vi "Robot_Main.vi"() -> ()   [LabVIEW 2013]
uses:
  Support VIs/setpointCluster.ctl
  GainsTDef.ctl
  Support VIs/speeds.ctl
  Support VIs/messageTypes.ctl
  PolarCoordTdef.ctl
  StopTDef.ctl
  <vilib>/robotics/Starter Kit/2.0/9632 Host Interface/NI_Robotics_Starter Kit Host_9632_2.0.lvclass
  <vilib>/robotics/Starter Kit/Host Interface/NI_Robotics_Starter Kit Host.lvclass
panel:
  out "message data":variant
  in  "Polar Coord":T1
  out "message type":T2=enum."Setpoints"
  in  "Speeds":T3
  in  "GainsCluster":T4
  in  "STOP":bool
  in  "Setpoint Cluster":T5
  out "Modulus Setpoint Read":dbl
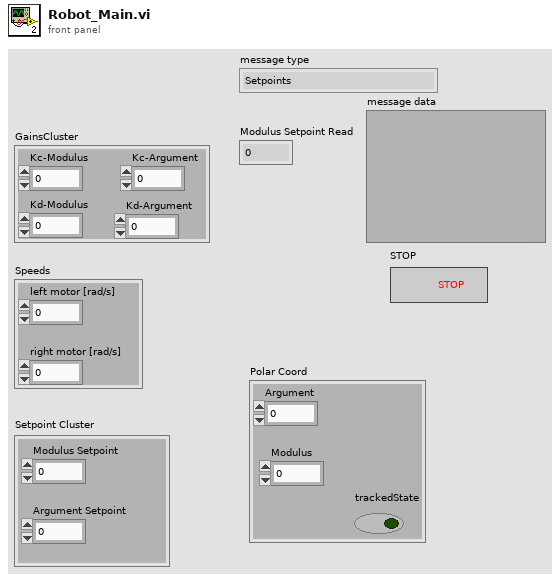
[diagram p1: front panel]
types:
  T1 = typedef "PolarCoordTdef.ctl" = cluster{"Argument":dbl, "Modulus":dbl, "trackedState":bool}
  T2 = typedef "messageTypes.ctl" = enum16{"Speeds", "Stop", "PolarCoordinates", "Gains", "Setpoints"}
  T3 = typedef "speeds.ctl" = cluster{"left motor [rad/s]":dbl, "right motor [rad/s]":dbl}
  T4 = typedef "GainsTDef.ctl" = cluster{"Kc-Modulus":dbl, "Kd-Modulus":dbl, "Kc-Argument":dbl, "Kd-Argument":dbl}
  T5 = typedef "setpointCluster.ctl" = cluster{"Modulus Setpoint":dbl, "Argument Setpoint":dbl}
  T6 = typedef "StopTDef.ctl" = cluster{"stop":bool}
  T7 = typedef "Messages.ctl" = cluster{"message data":variant, "message type":T2}
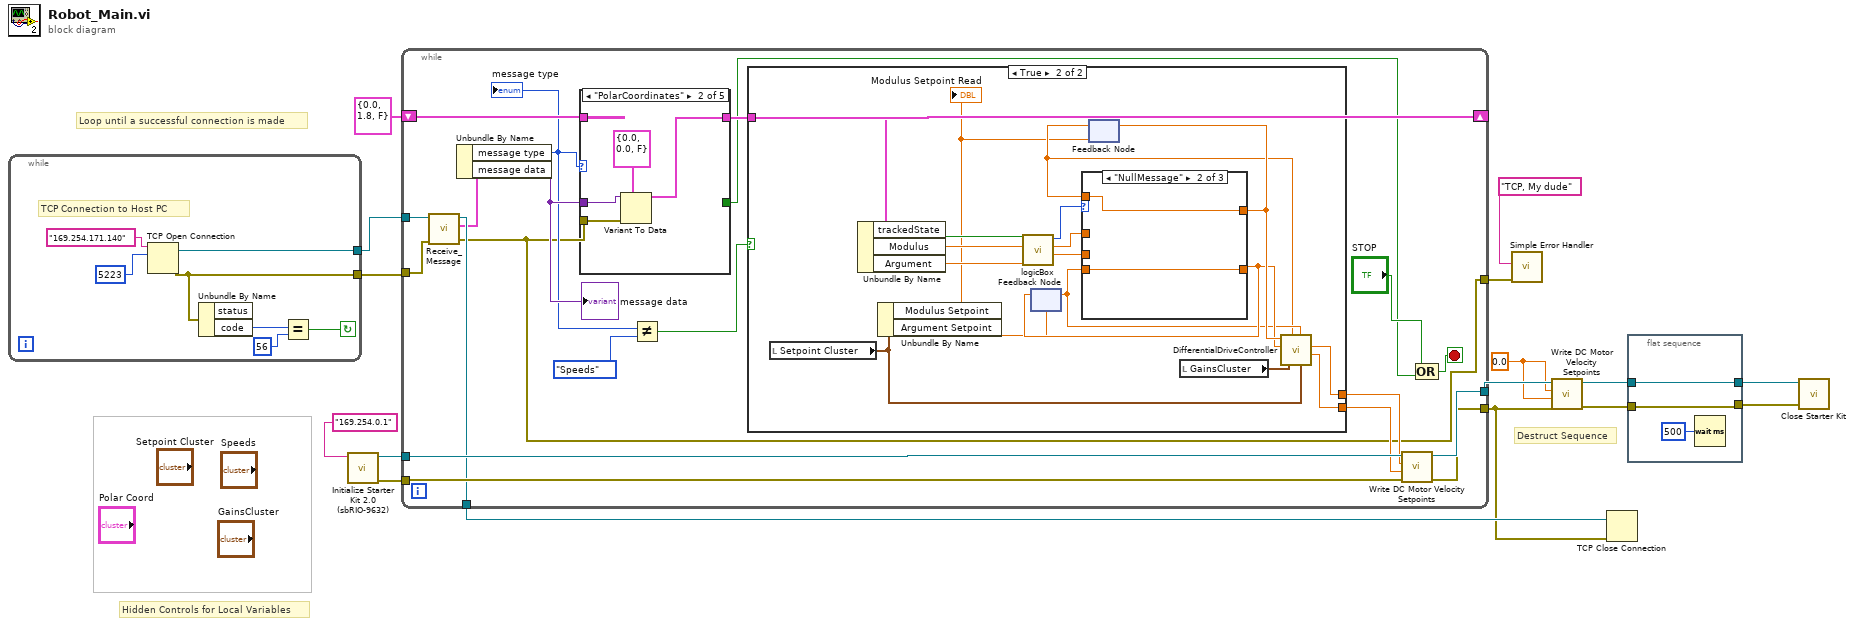
[diagram p0: block diagram]
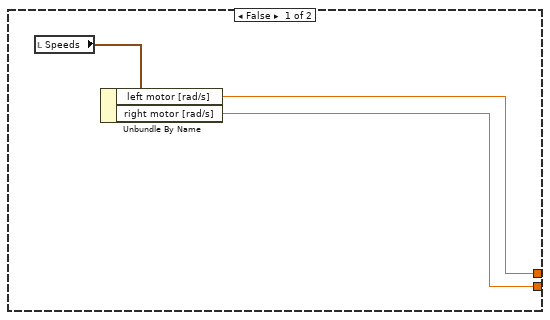
[diagram p2: hidden frame]
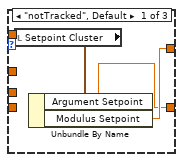
[diagram p3: hidden frame]
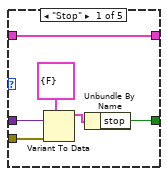
[diagram p5: hidden frame]
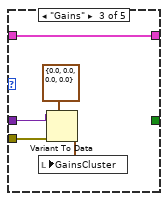
[diagram p6: hidden frame]
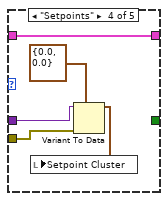
[diagram p7: hidden frame]
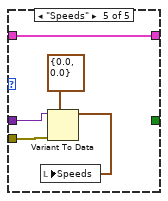
[diagram p8: hidden frame]
diagram:
  w13 = 0.0
  # "Hidden Controls for Local Variables"
  # "Loop until a successful connection is made"
  # "Destruct Sequence"
  n1 = while {
    tunnel: [w23] -> w6
    tunnel: [w20] -> w7
    stop <- w17 continue-if-true
    # "TCP Connection to Host PC"
    n2 = TCP Open Connection(address="169.254.171.140", remote port or service name=u16 5223) -> (connection ID=w23:refnum<k5>, error out=w20:errorcluster)  [unwired: 3 in]
    n3 = Unbundle By Name(w20) -> ("code"=w19:i32)  [unwired: 1 out]
    n4 = Equal?(x=w19, y=56) -> (x = y?=w17:bool)
  }
  n5 = call <vilib>:"Initialize Starter Kit 2.0 (sbRIO-9632).vi"("IP address (\"\")"="169.254.0.1" ("IP address (\"\")")) -> ("error out"=w15:errorcluster, "FPGA starter kit host 2.0 out"=w16:refnum<class "NI_Robotics_Starter Kit Host_9632_2.0.lvclass">)  [unwired: 9 in]
  n6 = while {
    tunnel: w16 -> [w43]
    tunnel: w15 -> [w34]
    tunnel: w7 -> [w39]
    tunnel: [w42] -> w14
    tunnel: [w41] -> w3
    tunnel: w6 -> [w40]
    shift-right: [w38] -> _
    shift-left: T1 {"Argument"=0.0, "Modulus"=1.8, "trackedState"=FALSE} ("Polar Coord") -> [w37]
    tunnel: [w33] -> w4
    tunnel: [w25] -> w2
    stop <- w27 stop-if-true
    n7 = call "Receive_Message.vi"("error in (no error)"=w39, "connection ID IN"=w40) -> ("error out (no error)"=w25:errorcluster, "msg OUT"=w31:T7, "connection ID OUT"=w33:refnum<k5>)  [unwired: 7 in]
    n8 = Unbundle By Name(w31) -> ("message type"=w29:T2, "message data"=w30:variant)
    "message type" <- w29
    "message data" <- w30
    n9 = case shown="\"PolarCoordinates\"" w29 {
      tunnel: w25 -> [w75 w79 w84 w89 w93]
      tunnel: [w73 w78 w83 w88 w95] -> w38
      tunnel: w37 -> [w73 _ w83 w88 w95]
      tunnel: w30 -> [w72 w77 w81 w86 w91]
      tunnel: [w71 _ _ _ _] -> w24
      frame "Stop" {
        n10 = Variant To Data(error in=w75, type=T6 {"stop"=FALSE}, Variant=w72) -> (data=w74:T6)  [unwired: 1 out]
        n11 = Unbundle By Name(w74) -> ("stop"=w71:bool)
      }
      frame "PolarCoordinates" {
        n12 = Variant To Data(error in=w79, type=T1 {"Argument"=0.0, "Modulus"=0.0, "trackedState"=FALSE} ("Polar Coord"), Variant=w77) -> (data=w78:T1)  [unwired: 1 out]
      }
      frame "Gains" {
        n13 = Variant To Data(error in=w84, type=T4 {"Kc-Modulus"=0.0, "Kd-Modulus"=0.0, "Kc-Argument"=0.0, "Kd-Argument"=0.0} ("GainsCluster"), Variant=w81) -> (data=w82:T4)  [unwired: 1 out]
        n14 = local write "GainsCluster"(w82) -> ()
      }
      frame "Setpoints" {
        n15 = Variant To Data(error in=w89, type=T5 {"Modulus Setpoint"=0.0, "Argument Setpoint"=0.0} ("Setpoint Cluster"), Variant=w86) -> (data=w87:T5)  [unwired: 1 out]
        n16 = local write "Setpoint Cluster"(w87) -> ()
      }
      frame "Speeds" {
        n17 = Variant To Data(error in=w93, type=T3 {"left motor [rad/s]"=0.0, "right motor [rad/s]"=0.0} ("Speeds"), Variant=w91) -> (data=w92:T3)  [unwired: 1 out]
        n18 = local write "Speeds"(w92) -> ()
      }
    }
    n19 = Not Equal?(x=w29, y=messageTypes."Speeds") -> (x != y?=w32:bool)
    n20 = case shown="True" w32 {
      tunnel: w38 -> [_ w63]
      tunnel: [w45 w56] -> w36
      tunnel: [w44 w55] -> w35
      frame False {
        n21 = local read "Speeds"() -> (w46:T3)
        n22 = Unbundle By Name(w46) -> ("left motor [rad/s]"=w45:dbl, "right motor [rad/s]"=w44:dbl)
      }
      frame True {
        n23 = local read "Setpoint Cluster"() -> (w48:T5)
        n24 = Unbundle By Name(w63) -> ("trackedState"=w62:bool, "Modulus"=w61:dbl, "Argument"=w60:dbl)
        n25 = Unbundle By Name(w48) -> ("Modulus Setpoint"=w49:dbl, "Argument Setpoint"=w50:dbl)
        "Modulus Setpoint Read" <- w49
        n26 = call "logicBox.vi"("Arg"=w60, "Mod"=w61, "TrackState"=w62) -> ("Arg"=w57:dbl, "Mod"=w58:dbl, "State"=w59:enum16{"notTracked", "NullMessage", "OK"})  [unwired: 6 in]
        n27 = feedback #1(w50) -> (w52:dbl)
        n28 = feedback #2(w49) -> (w51:dbl)
        n29 = case shown="\"NullMessage\"" w59 {
          tunnel: [w65 w67 w69] -> w53
          tunnel: [w66 w68 w70] -> w54
          tunnel: w58 -> [_ _ w70]
          tunnel: w57 -> [_ _ w69]
          tunnel: w51 -> [_ w68 _]
          tunnel: w52 -> [_ w67 _]
          frame "notTracked", Default {
            n30 = local read "Setpoint Cluster"() -> (w64:T5)
            n31 = Unbundle By Name(w64) -> ("Argument Setpoint"=w65:dbl, "Modulus Setpoint"=w66:dbl)
          }
          frame "NullMessage" {
          }
          frame "OK" {
          }
        }
        n32 = feedback-in #1(w53) -> ()
        n33 = feedback-in #2(w54) -> ()
        n34 = local read "GainsCluster"() -> (w47:T4)
        n35 = call "DifferentialDriveController.vi"("Setpoint Cluster"=w48, "prevArgIn"=w52, "GainsCluster"=w47, "prevModIn"=w51, "ArgIn"=w53, "ModIn"=w54) -> ("right motor out"=w55:dbl, "left motor out"=w56:dbl)  [unwired: 4 in]
      }
    }
    n36 = call <vilib>:"Write DC Motor Velocity Setpoints.vi"("error in (no error)"=w34, "right motor ccw velocity (rad/s)"=w35, "left motor ccw velocity (rad/s)"=w36, "starter kit host in"=w43) -> ("error out"=w41:errorcluster, "starter kit host out"=w42:refnum<class "NI_Robotics_Starter Kit Host_9632_2.0.lvclass">)  [unwired: 6 in]
    n37 = Compound Arithmetic op=OR("STOP", w24) -> (w27:bool)
  }
  n38 = call <vilib>:"Simple Error Handler.vi"("error source (\" \")"="TCP, My dude" ("error source (\" \")"), "error in (no error)"=w2) -> ()  [unwired: 3 in, 5 out]
  n39 = call <vilib>:"Write DC Motor Velocity Setpoints.vi"("error in (no error)"=w3, "right motor ccw velocity (rad/s)"=w13, "left motor ccw velocity (rad/s)"=w13, "starter kit host in"=w14) -> ("error out"=w11:errorcluster, "starter kit host out"=w12:refnum<class "NI_Robotics_Starter Kit Host_9632_2.0.lvclass">)  [unwired: 6 in]
  n40 = TCP Close Connection(connection ID=w4, error in (no error)=w3) -> ()  [unwired: 1 in, 2 out]
  n41 = flat-sequence {
    tunnel: w12 -> [w97]
    tunnel: w11 -> [w96]
    tunnel: [w97] -> w10
    tunnel: [w96] -> w9
    frame #0 {
      n42 = Wait (ms)(milliseconds to wait=u32 500) -> ()  [unwired: 1 out]
    }
  }
  n43 = call-dynamic "Close Starter Kit.vi"("error in (no error)"=w9, "starter kit host in"=w10) -> ()  [unwired: 9 in, 1 out]
